vi "hidSPD Read Multi Reports.vi"(8 "error in (no error)":errorcluster, 11 "spdDevSessions in":T2[](array[typedef])) -> (0 "error out":errorcluster, 2 "spd Reports":T1[](array[typedef]), 3 "spdDevSessions out":T2[](array[typedef]))   [LabVIEW 2018, in "hidSPDLibForLabView.lvlib"]
uses:
  hidSPDLibForLabView.lvlib
  hidSPD Controls/hidSPD Device Session.ctl
  hidSPD Controls/hidSPD Simple Report.ctl
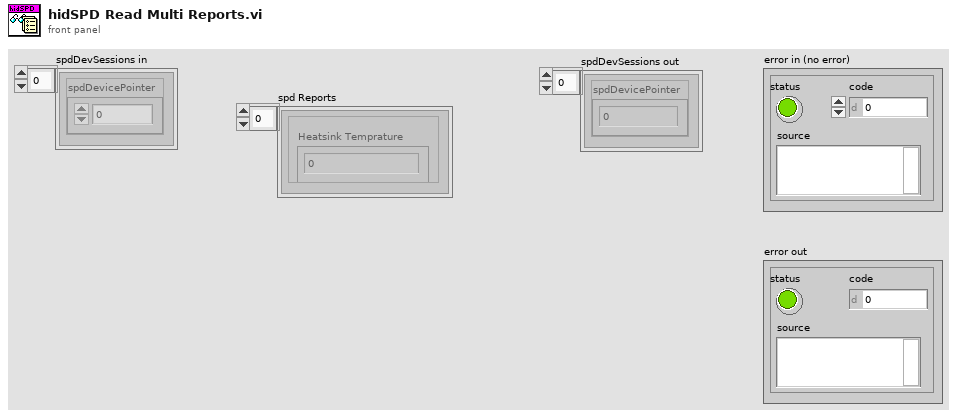
[diagram p1: front panel]
types:
  T1 = typedef "hidSPDLibForLabView.lvlib/hidSPD Simple Report.ctl" = cluster{"Heatsink Temprature":sgl, "Diod Temprature":sgl, "TEC-voltage":sgl, "Diod Bias":sgl, "RF Power":sgl, "Thermal used":sgl, "hv bias used":sgl, "hv code used":u16, "strobe code used":u16, "SPD number":u8, "SPD ready":u8}
  T2 = typedef "hidSPDLibForLabView.lvlib/hidSPD Device Session.ctl" = cluster{"spdDevicePointer":u64}
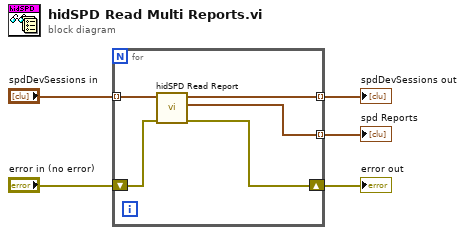
[diagram p0: block diagram]
diagram:
  n1 = for {
    tunnel: "spdDevSessions in" -> [w10] mode=indexing
    shift-right: [w8] -> w3
    shift-left: "error in (no error)" -> [w9]
    tunnel: [w7] -> w2 mode=indexing
    tunnel: [w6] -> w1 mode=indexing
    n2 = call "hidSPD Read Report.vi"("error in (no error)"=w9, "spdDevSession in"=w10) -> ("error out"=w8:errorcluster, "hidSPD Simple Report"=w6:T1, "spdDevSession out"=w7:T2)  [unwired: 7 in]
  }
  "error out" <- w3
  "spdDevSessions out" <- w2
  "spd Reports" <- w1
